vi "GLdrv_Read_TCPIP.vi"(0 "connection ID":refnum<k5>, 5 "Count":u32, 7 "Term(CrLf)":string="\r\n", 11 "error in (no error)":errorcluster, 12 "timeout ms":i32) -> (4 "connection ID out":refnum<k5>, 6 "data out":string, 15 "error out":errorcluster)   [LabVIEW 2017]
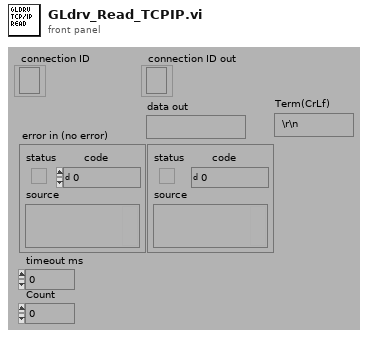
[diagram p1: front panel]
types:
  T1 = enum16{"Standard", "Buffered", "CRLF", "Immediate"}
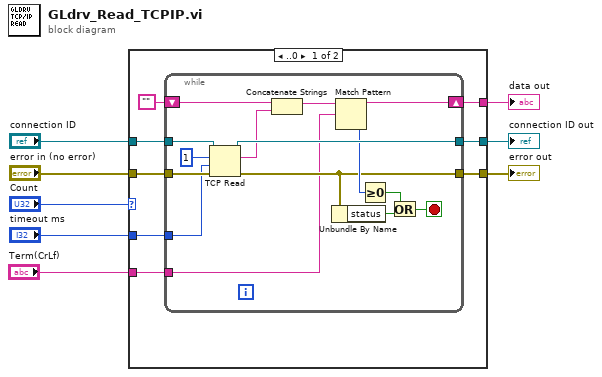
[diagram p0: block diagram]
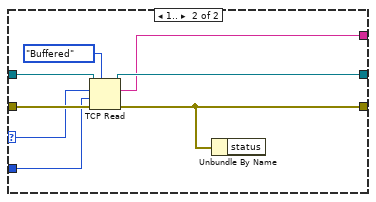
[diagram p2: hidden frame]
diagram:
  n1 = case shown="..0" "Count" {
    selector: "Count" -> [_ w33]
    tunnel: "error in (no error)" -> [w16 w39]
    tunnel: [w15 w38] -> w7
    tunnel: [w14 w34] -> w6
    tunnel: "connection ID" -> [w13 w37]
    tunnel: [w12 w36] -> w4
    tunnel: "timeout ms" -> [w11 w35]
    tunnel: "Term(CrLf)" -> [w9 _]
    frame ..0 {
      n2 = while {
        tunnel: w16 -> [w31]
        tunnel: [w22] -> w15
        tunnel: w13 -> [w30]
        tunnel: [w29] -> w12
        shift-right: [w25] -> w14
        shift-left: "" -> [w28]
        tunnel: w11 -> [w18]
        tunnel: w9 -> [w17]
        stop <- w19 stop-if-true
        n3 = TCP Read(connection ID=w30, bytes to read=1, error in (no error)=w31, 9:w18) -> (connection ID out=w29:refnum<k5>, data out=w27:string, error out=w22:errorcluster)  [unwired: 1 out]
        n4 = Concatenate Strings(w28, w27) -> (w24:string)
        n5 = Unbundle By Name(w22) -> ("status"=w21:bool)
        n6 = Match Pattern(string=w24, regular expression=w17) -> (before substring=w25:string, offset past match=w23:i32)  [unwired: 3 out]
        n7 = Greater Or Equal To 0?(x=w23) -> (x >= 0?=w20:bool)
        n8 = Or(x=w20, y=w21) -> (x .or. y?=w19:bool)
      }
    }
    frame 1.. {
      n9 = TCP Read(connection ID=w37, bytes to read=w33, error in (no error)=w39, 7:T1."Buffered" ("mode (standard)"), 9:w35) -> (connection ID out=w36:refnum<k5>, data out=w34:string, error out=w38:errorcluster)
      n10 = Unbundle By Name(w38) -> ()  [unwired: 1 out]
    }
  }
  "error out" <- w7
  "data out" <- w6
  "connection ID out" <- w4
